vi "Example Threshold.vi"() -> ()   [LabVIEW 2013]
uses:
  C:/tf/play/labview/Tinkerforge.dll
  Tinkerforge.dll
panel:
  in  "stop":bool
  out "callback counter":i32
  out "last current (mA)":sgl
  in  "uid":string="amb"
  in  "port":i32=4223
  in  "host":string="localhost"
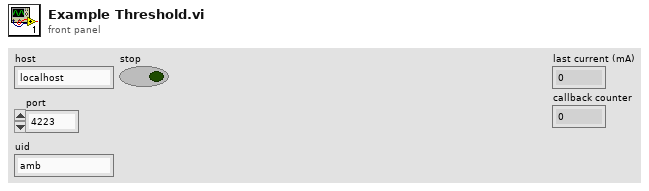
[diagram p1: front panel]
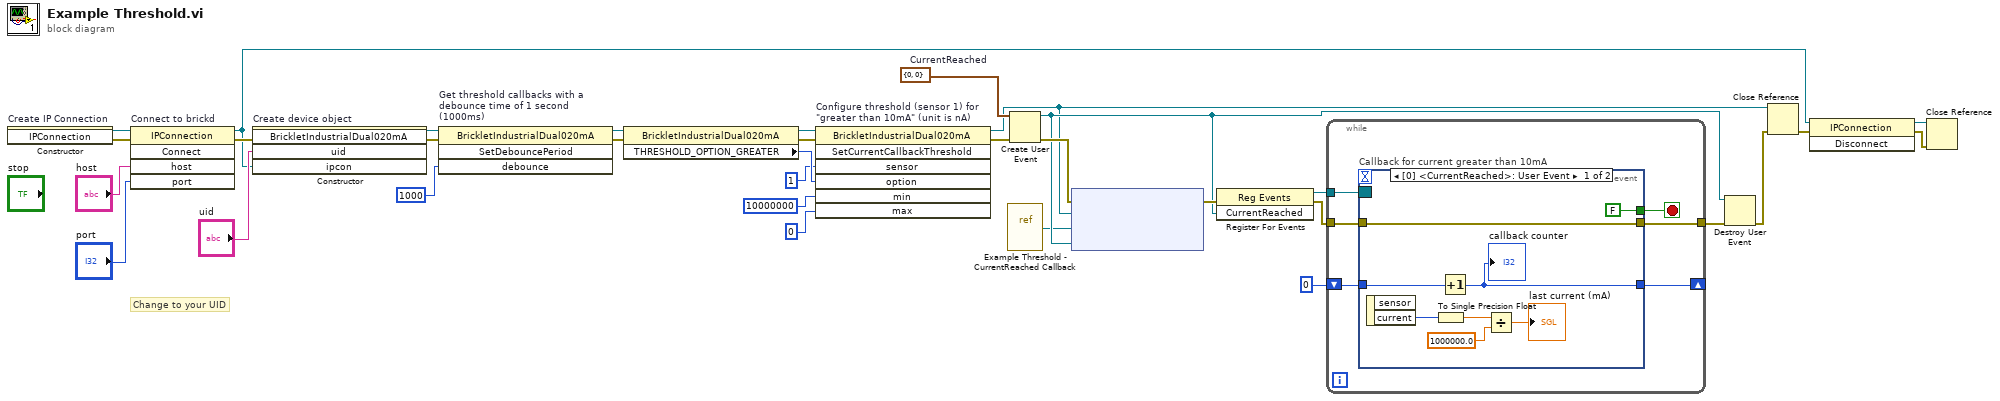
[diagram p0: block diagram]
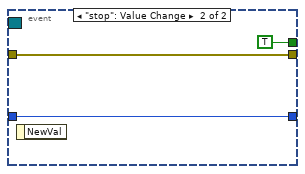
[diagram p2: hidden frame]
diagram:
  w17 = cluster{"sensor":u8, "current":i32} {"sensor"=0, "current"=0}  # CurrentReached
  # "Change to your UID"
  n1 = constructor on="Create IP Connection" class="IPConnection"() -> (reference out=w33:refnum<k24>, error out=w5:errorcluster)  [unwired: 3 in, 1 out]
  n2 = invoke on="Connect to brickd" class="IPConnection" method="Connect"(reference=w33, error in=w5, "host"="host", "port"="port") -> (reference out=w26:refnum<k24>, error out=w29:errorcluster)  [unwired: 1 in, 3 out]
  n3 = constructor on="Create device object" class="BrickletIndustrialDual020mA"(error in=w29, "uid"="uid", "ipcon"=w26) -> (reference out=w15:refnum<k24>, error out=w16:errorcluster)  [unwired: 2 in, 3 out]
  n4 = invoke on="Get threshold callbacks with a\ndebounce time of 1 second\n(1000ms)" class="BrickletIndustrialDual020mA" method="SetDebouncePeriod"(reference=w15, error in=w16, "debounce"=i64 1000 ("period")) -> (reference out=w9:refnum<k24>, error out=w11:errorcluster)  [unwired: 1 in, 2 out]
  n5 = property class="BrickletIndustrialDual020mA"(reference=w9, error in=w11) -> (reference out=w8:refnum<k24>, error out=w10:errorcluster, "THRESHOLD_OPTION_GREATER"=w2:u16)
  n6 = invoke on="Configure threshold (sensor 1) for\n\"greater than 10mA\" (unit is nA)" class="BrickletIndustrialDual020mA" method="SetCurrentCallbackThreshold"(reference=w8, error in=w10, "sensor"=u8 1, "option"=w2, "min"=10000000, "max"=0) -> (reference out=w13:refnum<k24>, error out=w12:errorcluster)  [unwired: 1 in, 5 out]
  n7 = vi-ref "Example Threshold - CurrentReached Callback.vi"() -> ("vi reference"=w6:refnum<vi>)
  n8 = Create User Event(user event datatype=w17, error in=w12) -> (user event=w19:refnum<user-event>, error out=w24:errorcluster)
  n9 = node ("Register Event Callback")(w24, w13, w6, w19) -> (w23:errorcluster)  [unwired: 1 in, 1 out]
  n10 = register-events(error in=w23, w19) -> (reference out=w22:refnum<event-registration>, error out=w20:errorcluster)  [unwired: 1 in]
  n11 = while {
    tunnel: w22 -> [w39]
    tunnel: [w38] -> w21
    tunnel: w20 -> [w37]
    shift-right: [w35] -> _
    shift-left: 0 -> [w36]
    stop <- w34 stop-if-true
    n12 = event "Callback for current greater than 10mA" shown="[0] <CurrentReached>: User Event" {
      selector: w39 -> [_ _]
      dyn-events: _ -> [_ _]
      timeout: _ -> [_ _]
      tunnel: [w44 w49] -> w38
      tunnel: w37 -> [w44 w49]
      tunnel: w36 -> [w42 w48]
      tunnel: [w41 w48] -> w35
      tunnel: [FALSE TRUE] -> w34
      event User Event {
        n13 = event-data() -> ("current"=w45:i32)  [unwired: 1 in, 1 out]
        n14 = To Single Precision Float(number=w45) -> (single precision float=w46:sgl)
        n15 = Increment(x=w42) -> (x+1=w41:i32)
        "callback counter" <- w41
        n16 = Divide(x=w46, y=sgl 1000000.0) -> (x/y=→"last current (mA)":sgl)
      }
      event "stop": Value Change {
        n17 = event-data() -> ()  [unwired: 1 in, 1 out]
      }
    }
  }
  n18 = Destroy User Event(user event=w19, error in=w21) -> (error out=w18:errorcluster)
  n19 = Close Reference(reference=w13, error in (no error)=w18) -> (error out=w28:errorcluster)
  n20 = invoke class="IPConnection" method="Disconnect"(reference=w26, error in=w28) -> (reference out=w25:refnum<k24>, error out=w27:errorcluster)  [unwired: 1 in, 1 out]
  n21 = Close Reference(reference=w25, error in (no error)=w27) -> ()  [unwired: 1 out]
